vi "sub_DO-relay-onoff.vi"(7 "onoff":bool=TRUE, 11 "현재채널번호":u8) -> ()   [LabVIEW 2019]
panel:
  in  "dt":u32=200
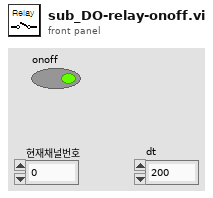
[diagram p1: front panel]
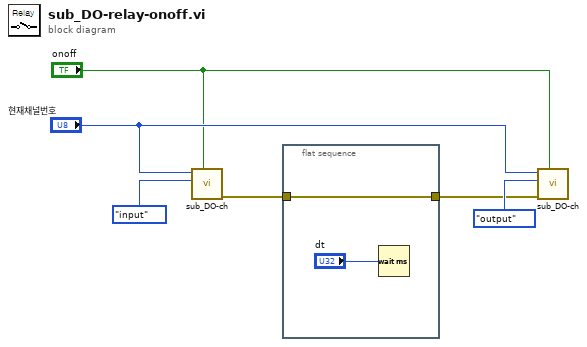
[diagram p0: block diagram]
diagram:
  n1 = call "sub_DO-ch.vi"("onoff"="onoff", "pos"=enum16{"input", "output"}."input", "현재채널번호"="현재채널번호") -> ("error out"=w2:errorcluster)  [unwired: 8 in]
  n2 = flat-sequence {
    tunnel: w2 -> [w8]
    tunnel: [w8] -> w1
    frame #0 {
      n3 = Wait (ms)(milliseconds to wait="dt") -> ()  [unwired: 1 out]
    }
  }
  n4 = call "sub_DO-ch.vi"("onoff"="onoff", "error in"=w1, "pos"=enum16{"input", "output"}."output", "현재채널번호"="현재채널번호") -> ()  [unwired: 7 in, 1 out]
